vi "set trigger.vi"(8 "error in (no error)":errorcluster, 11 "Cascade in":refnum<class "Cascade.lvclass">) -> (0 "error out":errorcluster, 3 "Cascade out":refnum<class "Cascade.lvclass">)   [LabVIEW 2012, in "Cascade.lvclass"]
uses:
  Cascade.lvclass
  Cascade.lvclass/Cascade.ctl
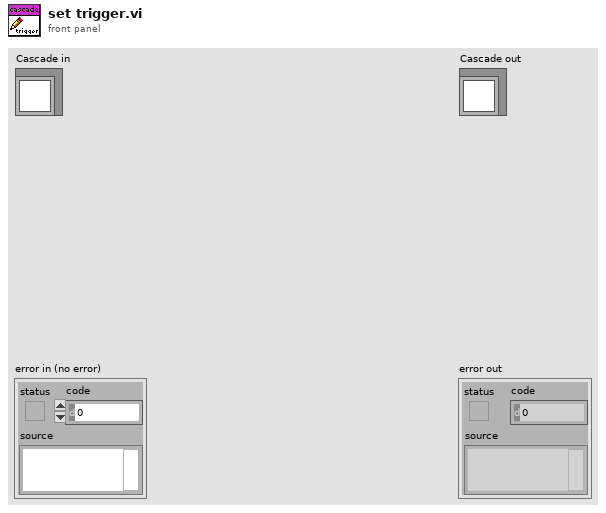
[diagram p1: front panel]
types:
  T1 = typedef "Cascade.lvclass/timing mode.ctl" = u32
  T2 = typedef "Cascade.lvclass/Trigger edge.ctl" = u32
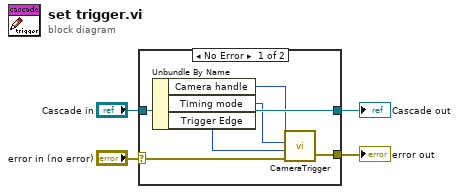
[diagram p0: block diagram]
diagram:
  n1 = case shown="No Error" "error in (no error)" {
    selector: "error in (no error)" -> [w10 w12]
    tunnel: [w9 w12] -> w3
    tunnel: [w8 w11] -> w1
    tunnel: "Cascade in" -> [w8 w11]
    frame No Error {
      n2 = Unbundle By Name(w8) -> ("Camera handle"=w7:u32, "Timing mode"=w6:T1, "Trigger Edge"=w5:T2)
      n3 = call <userlib>:"CameraTrigger.vi"("error in"=w10, "Trigger Edge"=w5, "Timing Mode"=w6, "Camera Handle"=w7) -> ("error out"=w9:errorcluster)  [unwired: 1 out]
    }
    frame Error {
    }
  }
  "error out" <- w3
  "Cascade out" <- w1
